vi "day 6 task 1 and 2.vi"() -> ()   [LabVIEW 2019]
panel:
  out "Last N char (buffer)":string[](array[string])
  out "position of first start of packet marker":i32
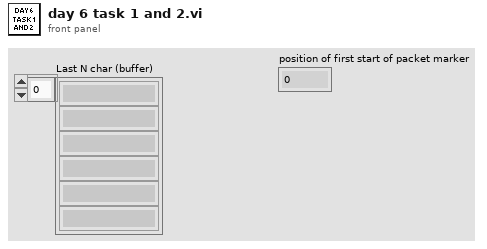
[diagram p1: front panel]
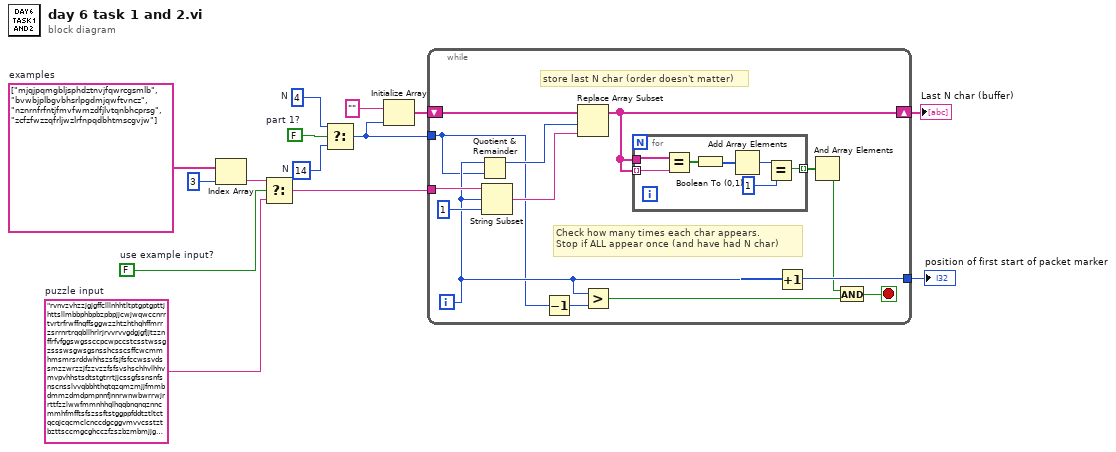
[diagram p0: block diagram]
diagram:
  w1 = 14  # N
  w4 = FALSE  # part 1?
  w2 = 4  # N
  w12 = string[] ["mjqjpqmgbljsphdztnvjfqwrcgsmlb", "bvwbjplbgvbhsrlpgdmjqwftvncz", "nznrnfrfntjfmvfwmzdfjlvtqnbhcprsg", "zcfzfwzzqfrljwzlrfnpqdbhtmscgvjw"]  # examples
  w13 = FALSE  # use example input?
  w14 = "rvnvzvhzzjgjgffclllnhhtltptgptgpttjhttsllmbbphbpbzpbpjjcwjwqwccnrrtvrtrfrwffnqffsggwzzhtzhthqhffmrrzsrrnrtrqqbllhrlrjrvvrvvgdgjgfjjtzznffrfvfggswgssccpcwpccstcsstwssgzssswsgwsgsnsshcsscsffcwcmmhmsmrsrddwhhszsfsjfsfccwssvdssmzzwrzzjfzzvzzfsfsvshschhvlhhvmvpvhhstsdtstgtrrtjjcssgfssnsnfsnscnsslvvqbbhthqtqzqmzmjjfmmbdmmzdmdpmpnnfjnnrwnwbwrrwjrrttfzzlwwfmmnhhqlhqqbnqnqznncmmhfmfftsfszssftstggppfddtztltctqcqjcqcmclcnccdgcggvmvvcsstztbzttsccmgcghcczfzszbzmbmjjggsqgghbhjjhhrrjljmllczlzzqssjfjqfjfmfdfgffczfzwwpfwpwbbftbffplphhfcftctlcclhlnlhnhlhnhqnhhjbjmmtpmmlsmllvhhjghhmzzwpzprrjrzzvrvcvqvssgssnccmgm..."  # puzzle input
  n1 = Index Array(array=w12, index=3) -> (element=w11:string)
  n2 = Select(t=w11, s=w13, f=w14) -> (s? t:f=w10:string)
  n3 = Select(t=w2, s=w4, f=w1) -> (s? t:f=w3:i32)
  n4 = Initialize Array("", w3) -> (w6:string[])
  n5 = while {
    tunnel: w10 -> [w28]
    tunnel: [w27] -> w7
    shift-right: [w19] -> w5
    shift-left: w6 -> [w22]
    tunnel: w3 -> [w15]
    i -> [w25]
    stop <- w23 stop-if-true
    # "Check how many times each char appears.\nStop if ALL appear once (and have had N char)"
    # "store last N char (order doesn't matter)"
    n6 = Quotient & Remainder(x=w25, y=w15) -> (x-y*floor(x/y)=w21:i32)  [unwired: 1 out]
    n7 = String Subset(string=w28, offset (0)=w25, length (rest)=1 ("length (rest)")) -> (substring=w20:string)
    n8 = Decrement(x=w15) -> (x-1=w16:i32)
    n9 = Replace Array Subset(array=w22, new element=w20, index=w21) -> (w19:string[])
    n10 = Greater?(x=w25, y=w16) -> (0:w24:bool)
    n11 = for {
      tunnel: w19 -> [w35] mode=indexing
      tunnel: w19 -> [w34]
      tunnel: [w29] -> w18 mode=indexing
      n12 = Equal?(x=w34, y=w35) -> (x = y?=w33:bool[])
      n13 = Boolean To (0,1)(Boolean=w33) -> (0, 1=w32:i16[])
      n14 = Add Array Elements(numeric array=w32) -> (sum=w31:i16)
      n15 = Equal?(x=w31, y=i16 1) -> (x = y?=w29:bool)
    }
    n16 = Increment(x=w25) -> (x+1=w27:i32)
    n17 = And Array Elements(Boolean array=w18) -> (logical AND=w17:bool)
    n18 = And(x=w17, y=w24) -> (x .and. y?=w23:bool)
  }
  "position of first start of packet marker" <- w7
  "Last N char (buffer)" <- w5
